vi "Bus Interface.vi"(0 "Oscillator":refnum<class "Oscillator.lvclass">, 1 "abort":bool, 5 "instruction":T2, 9 "input valid":bool) -> (6 "response":T1, 10 "done":bool, 14 "ready for input":bool)   [LabVIEW 2017, in "Oscillator.lvlib" / "Oscillator.lvclass"]
uses:
  Oscillator.lvclass
  <instrlib>/_niInstr/Instruction Framework/v1/FPGA/Interfaces/Address Space/Address Space Instruction.ctl
  <instrlib>/_niInstr/Instruction Framework/v1/FPGA/Typedefs/Response.ctl
  <instrlib>/_niInstr/Instruction Framework/v1/FPGA/Typedefs/niInstr Instruction Framework v1 FPGA.lvlib
  <instrlib>/_niInstr/Instruction Framework/v1/FPGA/Interfaces/Address Space/Address Space.lvclass
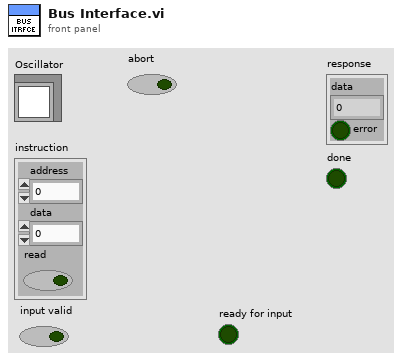
[diagram p1: front panel]
types:
  T1 = typedef "niInstr Instruction Framework v1 FPGA.lvlib/Response.ctl" = cluster{"data":u64, "error":bool}
  T2 = typedef "niInstr Instruction Framework Interfaces v1 FPGA.lvlib/Address Space.lvclass/Address Space Instruction.ctl" = cluster{"address":u32, "data":u64, "read":bool}
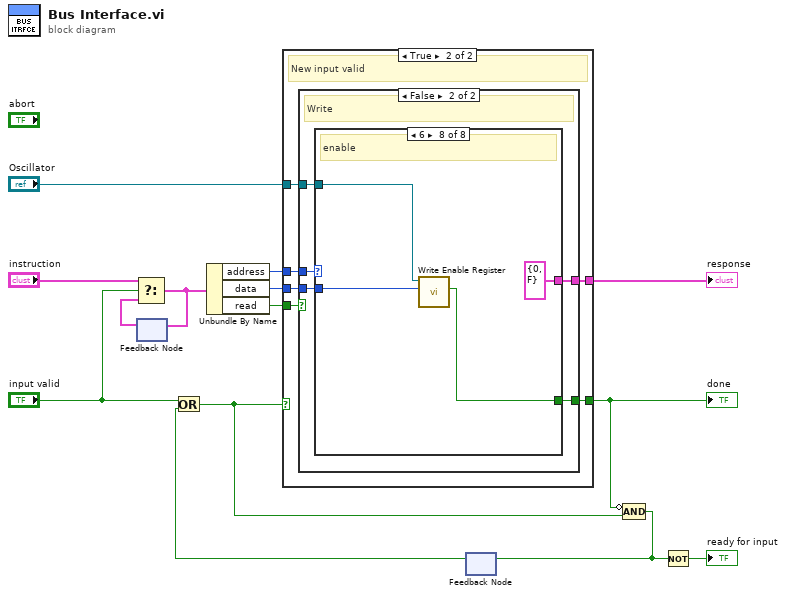
[diagram p0: block diagram]
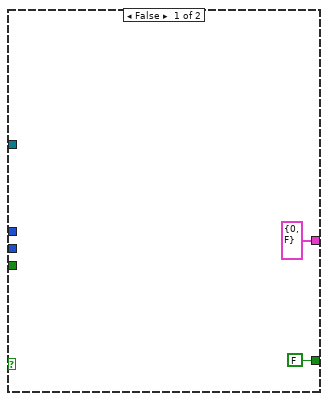
[diagram p2: hidden frame]
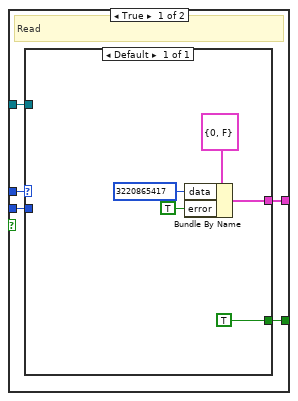
[diagram p3: hidden frame]
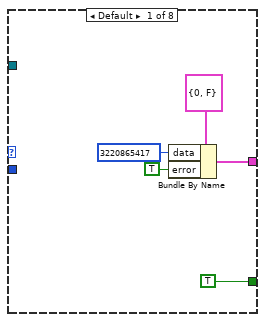
[diagram p4: hidden frame]
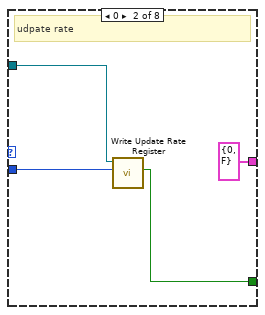
[diagram p5: hidden frame]
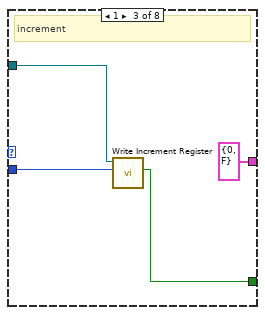
[diagram p6: hidden frame]
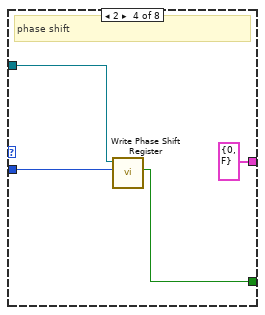
[diagram p7: hidden frame]
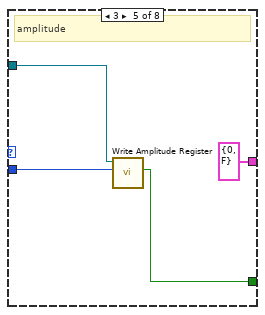
[diagram p8: hidden frame]
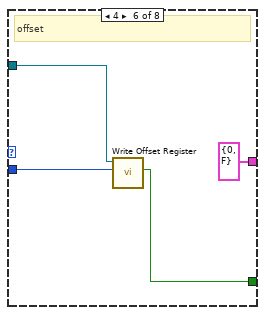
[diagram p9: hidden frame]
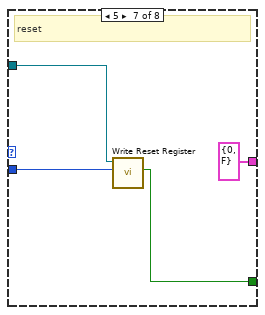
[diagram p10: hidden frame]
diagram:
  n1 = feedback #1() -> (w13:T2)  [unwired: 1 in]
  n2 = Select(t="instruction", s="input valid", f=w13) -> (s? t:f=w12:T2)
  n3 = feedback-in #1(w12) -> ()
  n4 = Unbundle By Name(w12) -> ("address"=w9:u32, "data"=w7:u64, "read"=w10:bool)
  n5 = feedback #2() -> (w3:bool)  [unwired: 1 in]
  n6 = Or(x="input valid", y=w3) -> (x .or. y?=w4:bool)
  n7 = case shown="True" w4 {
    tunnel: w10 -> [_ w22]
    tunnel: w9 -> [_ w21]
    tunnel: "Oscillator" -> [_ w20]
    tunnel: w7 -> [_ w19]
    tunnel: [T1 {"data"=0, "error"=FALSE} ("response") w18] -> w6
    tunnel: [FALSE w17] -> w5
    frame False {
    }
    frame True {
      # "New input valid"
      n8 = case shown="False" w22 {
        tunnel: w21 -> [w27 w37]
        tunnel: w20 -> [w26 w36]
        tunnel: w19 -> [w23 w33]
        tunnel: [w24 w34] -> w18
        tunnel: [w25 w35] -> w17
        frame True {
          # "Read"
          n9 = case shown="Default" w27 {
            tunnel: w26 -> [_]
            tunnel: [w29] -> w24
            tunnel: [TRUE] -> w25
            tunnel: w23 -> [_]
            frame Default {
              n10 = Bundle By Name(cluster=T1 {"data"=0, "error"=FALSE} ("response"), "data"=u64 3220865417, "error"=TRUE) -> (w29:T1)
            }
          }
        }
        frame False {
          # "Write"
          n11 = case shown="6" w37 {
            tunnel: w36 -> [_ w45 w49 w53 w57 w61 w65 w69]
            tunnel: [w39 T1 {"data"=0, "error"=FALSE} ("response") T1 {"data"=0, "error"=FALSE} ("response") T1 {"data"=0, "error"=FALSE} ("response") T1 {"data"=0, "error"=FALSE} ("response") T1 {"data"=0, "error"=FALSE} ("response") T1 {"data"=0, "error"=FALSE} ("response") T1 {"data"=0, "error"=FALSE} ("response")] -> w34
            tunnel: [TRUE w46 w50 w54 w58 w62 w66 w70] -> w35
            tunnel: w33 -> [_ w44 w48 w52 w56 w60 w64 w68]
            frame Default {
              n12 = Bundle By Name(cluster=T1 {"data"=0, "error"=FALSE} ("response"), "data"=u64 3220865417, "error"=TRUE) -> (w39:T1)
            }
            frame 0 {
              # "udpate rate"
              n13 = call "Write Update Rate Register.vi"("data"=w44, "Oscillator Address Space in"=w45) -> ("done"=w46:bool)  [unwired: 9 in]
            }
            frame 1 {
              # "increment"
              n14 = call "Write Increment Register.vi"("data"=w48, "Oscillator Address Space in"=w49) -> ("done"=w50:bool)  [unwired: 9 in]
            }
            frame 2 {
              # "phase shift"
              n15 = call "Write Phase Shift Register.vi"("data"=w52, "Oscillator Address Space in"=w53) -> ("done"=w54:bool)  [unwired: 9 in]
            }
            frame 3 {
              # "amplitude"
              n16 = call "Write Amplitude Register.vi"("data"=w56, "Oscillator Address Space in"=w57) -> ("done"=w58:bool)  [unwired: 9 in]
            }
            frame 4 {
              # "offset"
              n17 = call "Write Offset Register.vi"("data"=w60, "Oscillator Address Space in"=w61) -> ("done"=w62:bool)  [unwired: 9 in]
            }
            frame 5 {
              # "reset"
              n18 = call "Write Reset Register.vi"("data"=w64, "Oscillator Address Space in"=w65) -> ("done"=w66:bool)  [unwired: 9 in]
            }
            frame 6 {
              # "enable"
              n19 = call "Write Enable Register.vi"("data"=w68, "Oscillator Address Space in"=w69) -> ("done"=w70:bool)  [unwired: 9 in]
            }
          }
        }
      }
    }
  }
  "done" <- w5
  "response" <- w6
  n20 = Compound Arithmetic op=AND(invert w5, w4) -> (w2:bool)
  n21 = feedback-in #2(w2) -> ()
  n22 = Not(x=w2) -> (.not. x?=→"ready for input":bool)
